vi "Finalización_Turbi.vi"(0 "Refnum in":refnum<k21>, 5 "error in":errorcluster) -> (19 "error out":errorcluster)   [LabVIEW 2013]
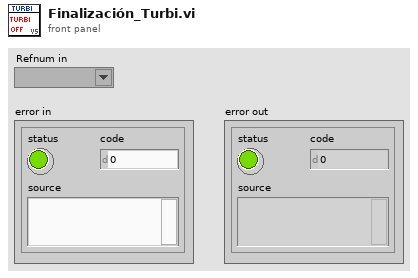
[diagram p1: front panel]
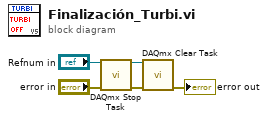
[diagram p0: block diagram]
diagram:
  n1 = call <vilib>:"DAQmx Stop Task.vi"("task/channels in"="Refnum in", "error in"="error in") -> ("task out"=w1:refnum<k21>, "error out"=w4:errorcluster)  [unwired: 12 in]
  n2 = call <vilib>:"DAQmx Clear Task.vi"("task in"=w1, "error in"=w4) -> ("error out"=→"error out":errorcluster)  [unwired: 13 in]
